vi "EMD8216 subnet mask set.vi"(9 "subnet_mask":u8[](array[numeric]), 11 "CardID":u32) -> (3 "error_code":u32)   [LabVIEW 2009, in "EMD8216_64.lvlib"]
doc: "EMD8216Status EMD8216_subnet_mask_set(u32 CardID,u8 subnet_mask[4]);"
uses:
  EMD8216_64.lvlib
  <userlib>/EMD8216_64/EMD8216_64.dll
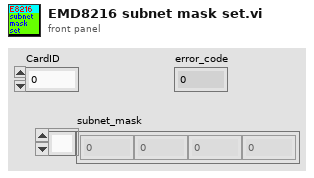
[diagram p1: front panel]
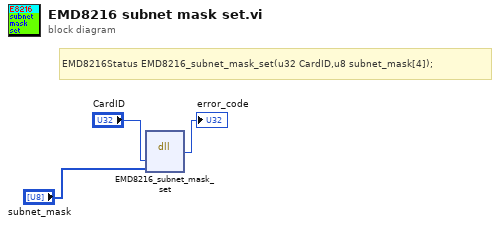
[diagram p0: block diagram]
diagram:
  # "EMD8216Status EMD8216_subnet_mask_set(u32 CardID,u8 subnet_mask[4]);"
  n1 = dll-call lib="C:/Program Files/National Instruments/LabVIEW 2017/user.lib/EMD8216_64/EMD8216_64.*" fn="EMD8216_subnet_mask_set"("CardID"="CardID", "subnet_mask"="subnet_mask") -> ("return type"=→"error_code":u32)  [unwired: 5 in, 2 out]
